vi "Chart Window.vi"() -> ()   [LabVIEW 2019]
uses:
  SubVIs/WSData.vi
panel:
  out "Waveform Chart":T1(graph)={"data[0]"=18.911298857159423, "data[1]"=59.99536966047508, "data[2]"=0.0, "data[3]"=0.0, "data[4]"=0.0, "data[5]"=0.0, "data[6]"=0.0, "data[7]"=0.0, "data[8]"=0.0}
  out "Error Out":errorcluster
  in  "Error In":errorcluster
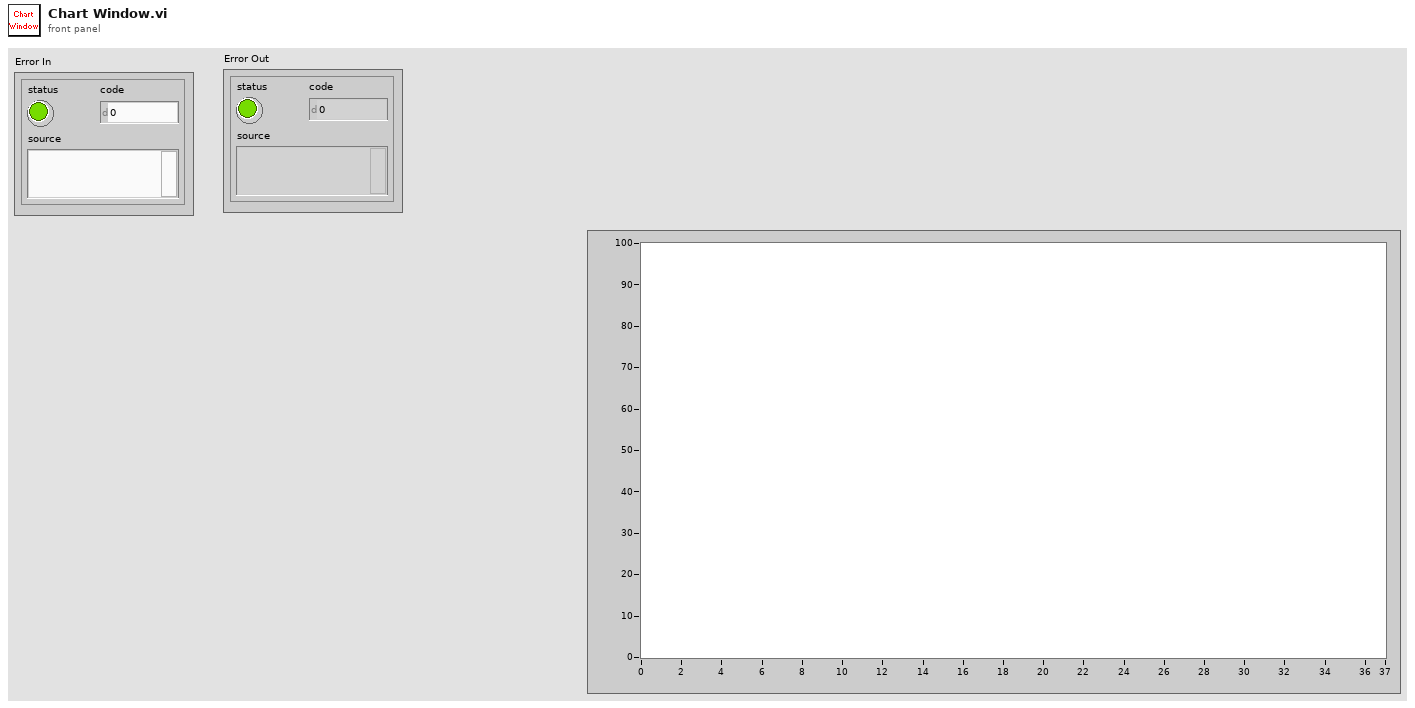
[diagram p1: front panel]
types:
  T1 = cluster{"data[0]":dbl, "data[1]":dbl, "data[2]":dbl, "data[3]":dbl, "data[4]":dbl, "data[5]":dbl, "data[6]":dbl, "data[7]":dbl, "data[8]":dbl}
  T2 = cluster{"data[0]":dbl, "data[1]":dbl, "data[2]":dbl, "data[3]":dbl, "data[4]":dbl, "data[5]":dbl, "data[6]":dbl, "data[7]":dbl, "data[8]":dbl}[]
  T3 = cluster{"DataEU[0]":dbl, "DataEU[1]":dbl, "DataEU[2]":dbl, "DataEU[3]":dbl, "DataEU[4]":dbl, "DataEU[5]":dbl, "DataEU[6]":dbl, "DataEU[7]":dbl, "DataEU[8]":dbl}
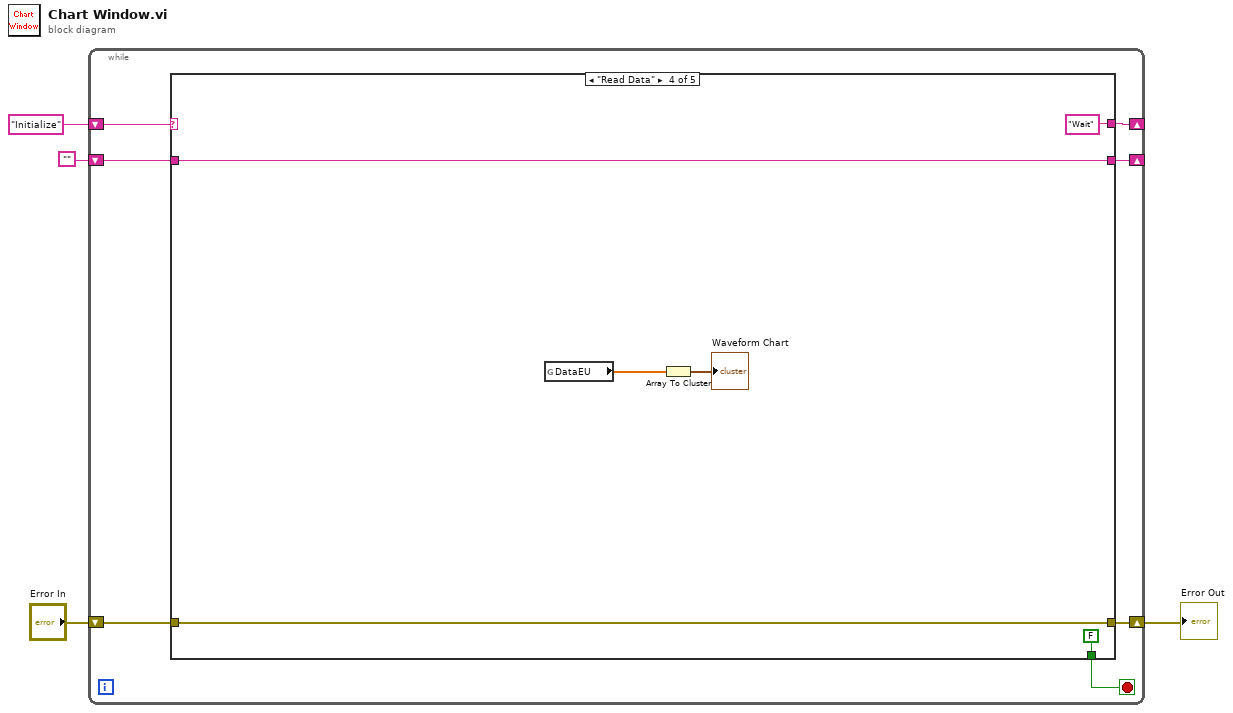
[diagram p0: block diagram]
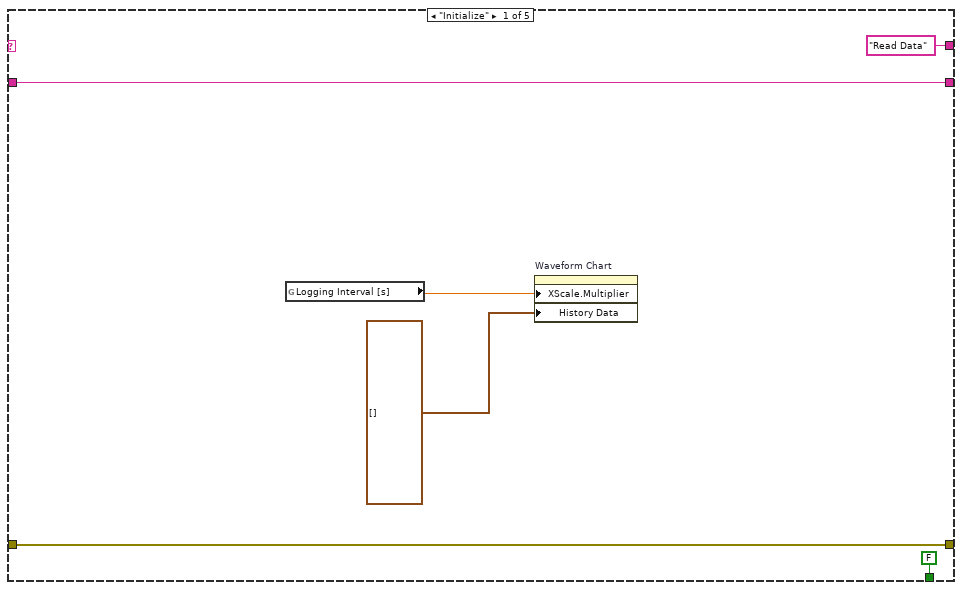
[diagram p2: hidden frame]
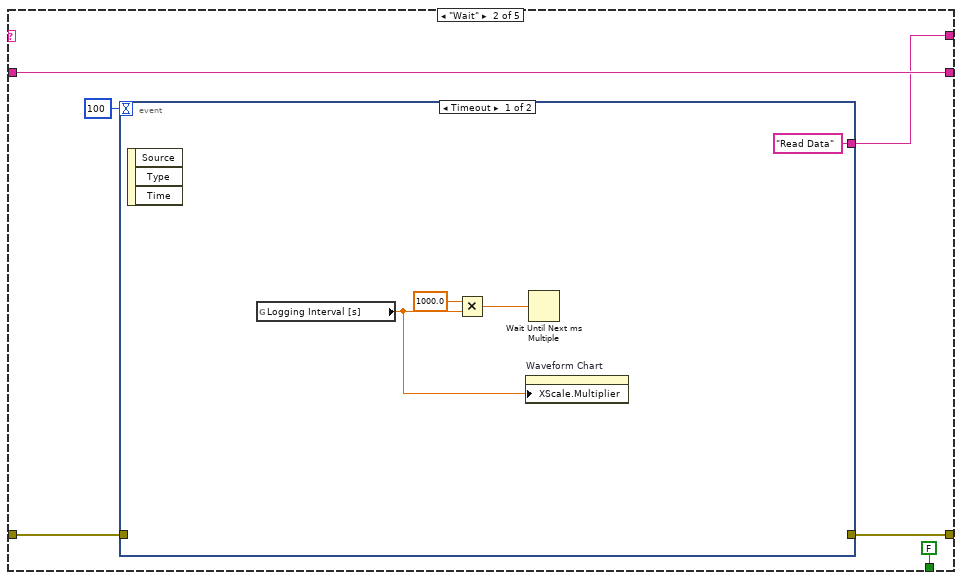
[diagram p3: hidden frame]
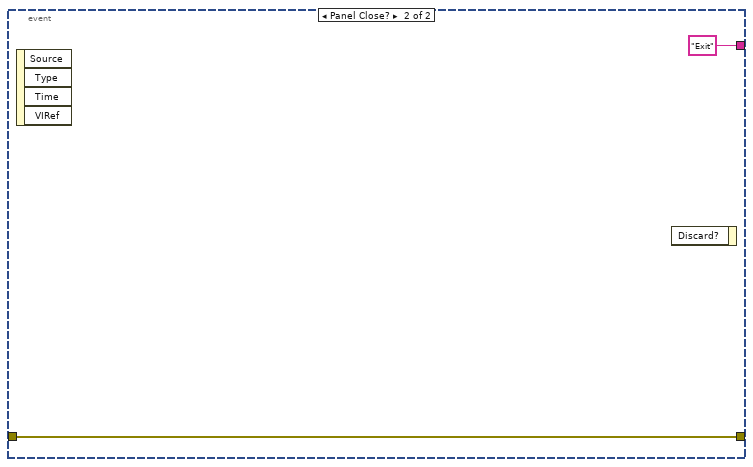
[diagram p4: hidden frame]
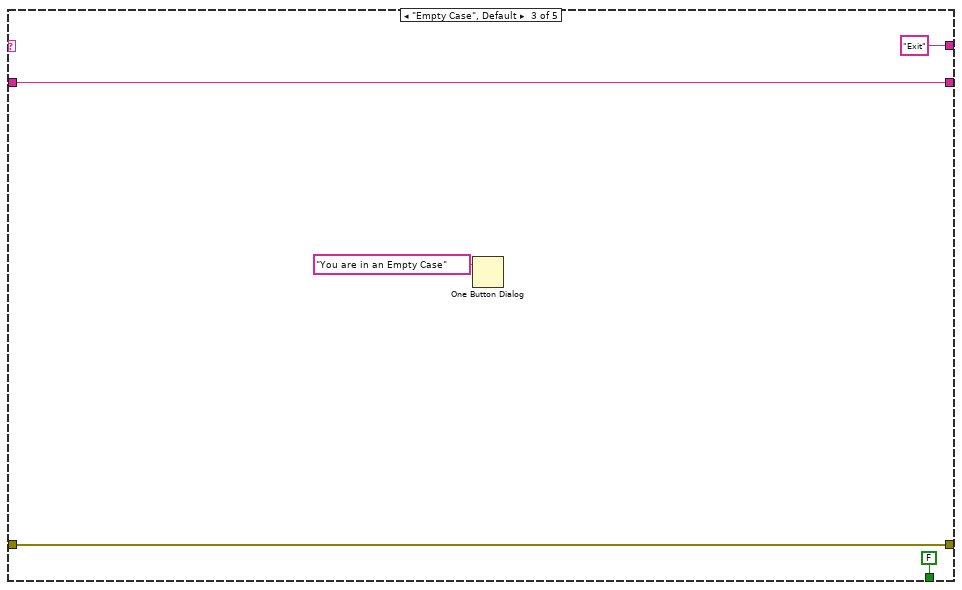
[diagram p5: hidden frame]
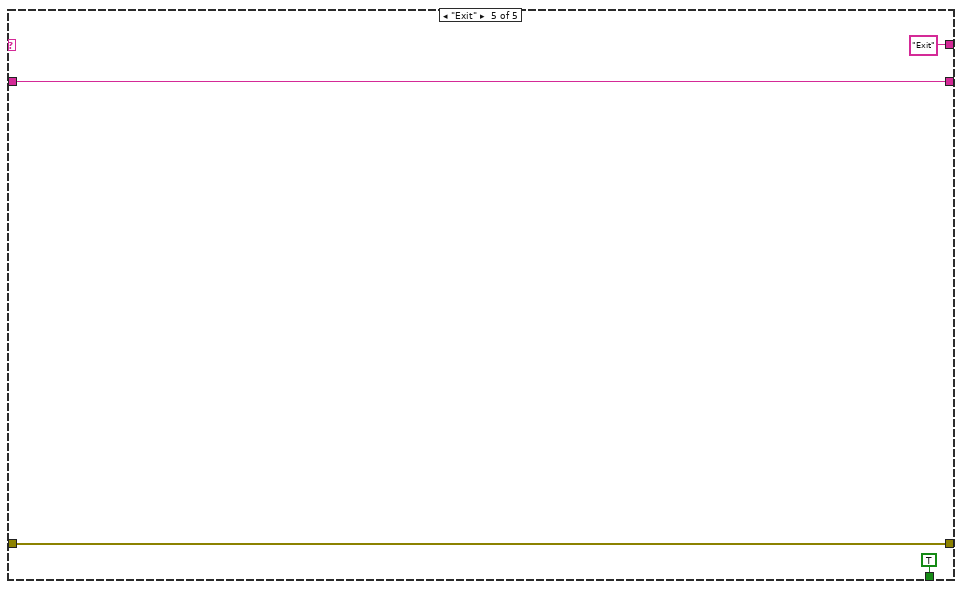
[diagram p6: hidden frame]
diagram:
  n1 = while {
    shift-right: [w7] -> _
    shift-left: "Initialize" ("key") -> [w11]
    shift-right: [w8] -> _
    shift-left: "" -> [w10]
    shift-right: [w5] -> w2
    shift-left: "Error In" -> [w9]
    stop <- w6 stop-if-true
    n2 = case shown="\"Read Data\"" w11 {
      tunnel: w10 -> [w14 w22 w31 w37 w44]
      tunnel: w9 -> [w15 w19 w32 w38 w41]
      tunnel: [w14 w22 w31 w37 w44] -> w8
      tunnel: ["Read Data" ("key") w21 "Exit" ("key") "Wait" ("key") "Exit" ("key")] -> w7
      tunnel: [FALSE FALSE FALSE FALSE TRUE] -> w6
      tunnel: [w15 w18 w32 w38 w41] -> w5
      frame "Initialize" {
        n3 = global read "WSData.vi" "Logging Interval [s]"() -> (w12:dbl)
        n4 = property on="Waveform Chart" class="WFChart (strict)"("XScale.Multiplier"=w12, "History Data"=T2 []) -> ()  [unwired: 2 in, 2 out]
      }
      frame "Wait" {
        n5 = event shown="[0] Timeout" {
          selector: _ -> [_ _]
          dyn-events: _ -> [_ _]
          timeout: 100 -> [_ _]
          tunnel: ["Read Data" ("key") "Exit" ("key")] -> w21
          tunnel: w19 -> [_ w28]
          tunnel: [_ w28] -> w18
          event Timeout {
            n6 = event-data() -> ()  [unwired: 1 in, 3 out]
            n7 = global read "WSData.vi" "Logging Interval [s]"() -> (w24:dbl)
            n8 = Multiply(x=1000.0, y=w24) -> (x*y=w25:dbl)
            n9 = property on="Waveform Chart" class="WFChart (strict)"("XScale.Multiplier"=w24) -> ()  [unwired: 2 in, 2 out]
            n10 = Wait Until Next ms Multiple(millisecond multiple=w25) -> ()  [unwired: 1 out]
          }
          event Panel Close? {
            n11 = event-data() -> ()  [unwired: 1 in, 4 out]
            n12 = event-data() -> ()  [unwired: 2 in, 1 out]
          }
        }
      }
      frame "Empty Case", Default {
        n13 = One Button Dialog(message="You are in an Empty Case") -> ()  [unwired: 1 in, 1 out]
      }
      frame "Read Data" {
        n14 = global read "WSData.vi" "DataEU"() -> (w36:dbl[])
        n15 = Array To Cluster(array=w36) -> (cluster=→"Waveform Chart":T3)
      }
      frame "Exit" {
      }
    }
  }
  "Error Out" <- w2
